vi "Set Channel Value Table.vi"(8 "Error In":errorcluster, 9 "Values":dbl[](array[numeric]), 10 "Names":string[](array[string]), 11 "Channel Ref In":T1 format="%.0x") -> (0 "Error Out":errorcluster, 3 "Channel Ref Out":T1=18446744073709551615 format="%.0x")   [LabVIEW 2023, in "Instrument Addon Shared.lvlib"]
uses:
  Instrument Addon Shared.lvlib
  <vilib>/NI VeriStand/Custom Device API/Custom Device Item Ref.ctl
  NationalInstruments.VeriStand.SystemStorage
  <vilib>/NI VeriStand/Custom Device API/Custom Device API.lvlib
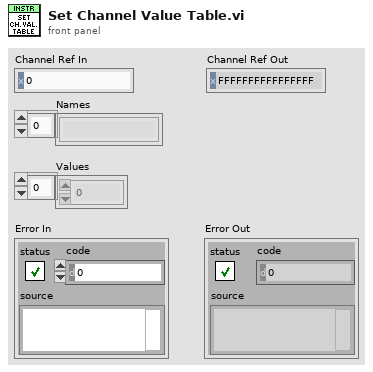
[diagram p1: front panel]
types:
  T1 = typedef "Custom Device API.lvlib/Custom Device Item Ref.ctl" = u64
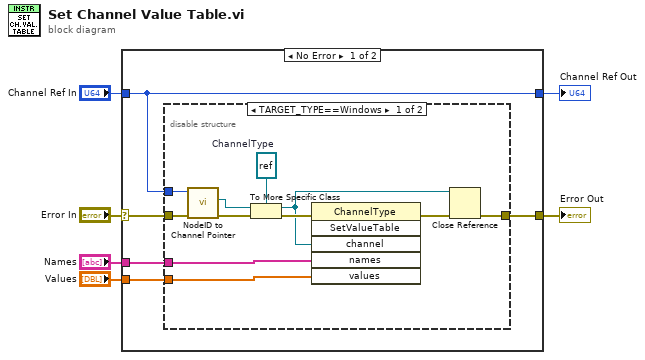
[diagram p0: block diagram]
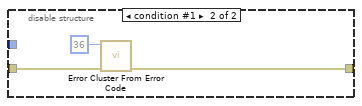
[diagram p2: hidden frame]
diagram:
  n1 = case shown="No Error" "Error In" {
    selector: "Error In" -> [w11 w27]
    tunnel: [w9 w27] -> w6
    tunnel: "Channel Ref In" -> [w10 w26]
    tunnel: [w10 w26] -> w4
    tunnel: "Names" -> [w8 _]
    tunnel: "Values" -> [w7 _]
    frame No Error {
      n2 = disable-structure shown="TARGET_TYPE==Windows" {
        disable-tunnel: w11 -> [w15 w25]
        disable-tunnel: w10 -> [w13 _]
        disable-tunnel: [w20 w24] -> w9
        disable-tunnel: w8 -> [w17 _]
        disable-tunnel: w7 -> [w18 _]
        frame condition #0 (active) {
          w19 = refnum<k24> refnum  # ChannelType
          n3 = call "NodeID to Channel Pointer.vi"("error in (no error)"=w15, "nodeID in"=w13) -> ("error out"=w14:errorcluster, "BaseNodeType out"=w12:refnum<k24>)  [unwired: 7 in, 1 out]
          n4 = To More Specific Class(target class=w19, reference=w12, error in=w14) -> (specific class reference=w16:refnum<k24>, error out=w22:errorcluster)
          n5 = invoke class="ChannelType" method="SetValueTable"(error in=w22, "channel"=w16, "names"=w17, "values"=w18) -> (error out=w21:errorcluster)  [unwired: 2 in, 5 out]
          n6 = Close Reference(reference=w16, error in (no error)=w21) -> (error out=w20:errorcluster)
        }
        frame condition #1 {
          n7 = call <vilib>:"Error Cluster From Error Code.vi"("error in (no error)"=w25, "error code (0)"=36) -> ("error out"=w24:errorcluster)  [unwired: 7 in]
        }
      }
    }
    frame Error {
    }
  }
  "Error Out" <- w6
  "Channel Ref Out" <- w4
